vi "Jacobian.vi"(8 "q2":dbl, 9 "q1":dbl, 11 "L":dbl) -> (2 "J":T1)   [LabVIEW 2019]
uses:
  <vilib>/Analysis/Matrix/Datatypes/RealMatrix.ctl
  <vilib>/Analysis/Matrix/NI_Matrix.lvlib
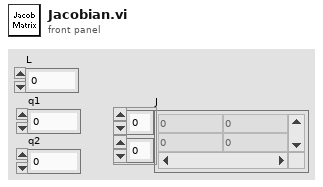
[diagram p1: front panel]
types:
  T1 = typedef "NI_Matrix.lvlib/RealMatrix.ctl" = dbl[][]
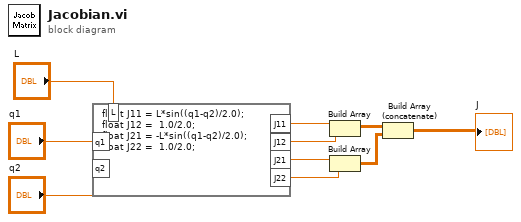
[diagram p0: block diagram]
diagram:
  n1 = formula code="float J11 = L*sin((q1-q2)/2.0);\nfloat J12 =  1.0/2.0;\nfloat J21 = -L*sin((q1-q2)/2.0);\nfloat J22 =  1.0/2.0;"("q2"="q2", "q1"="q1", "L"="L") -> ("J11"=w7:dbl, "J12"=w6:dbl, "J21"=w5:dbl, "J22"=w4:dbl)
  n2 = Build Array(w7, w6) -> (w3:T1)
  n3 = Build Array(w5, w4) -> (w2:T1)
  n4 = Build Array (concatenate)(w3, w2) -> (→"J":T1)
